vi "Filter Triggered.vi"(8 "error in (no error)":errorcluster, 10 "Assert Message":T1, 11 "Boolean Filter in":refnum<class "Boolean Filter.lvclass">) -> (0 "error out":errorcluster, 2 "Filtered":bool)   [LabVIEW 2018, in "Assert API Components.lvlib" / "Boolean Filter.lvclass"]
uses:
  Boolean Filter.lvclass
  Message Data.ctl
  Failure Actions.ctl
  Base Filter.lvclass
  Assert API Components.lvlib
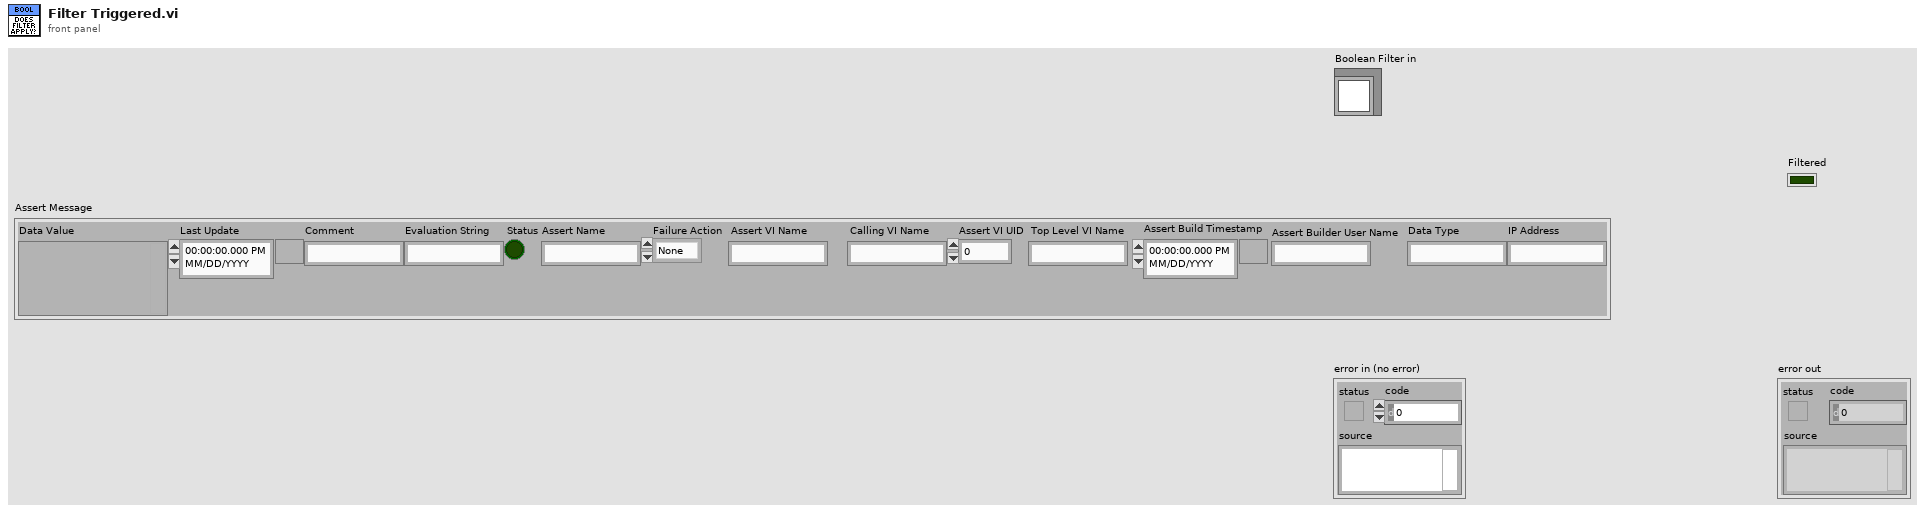
[diagram p1: front panel]
types:
  T1 = typedef "Assert API Components.lvlib/Message Data.ctl" = cluster{"Data Value":variant, "Last Update":timestamp, "Comment":string, "Evaluation String":string, "Status":bool, "Assert Name":string, "Failure Action":T2, "Assert VI Name":string, "Calling VI Name":string, "Assert VI UID":i32, "Top Level VI Name":string, "Assert Build Timestamp":timestamp, "Assert Builder User Name":string, "Data Type":string, "IP Address":string}
  T2 = typedef "Assert API Components.lvlib/Failure Actions.ctl" = enum16{"None", "Log To File", "Pause Execution", "Abort Execution"}
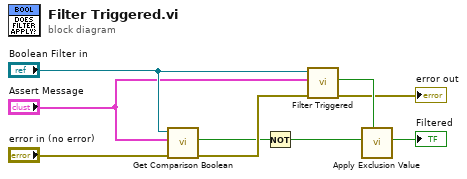
[diagram p0: block diagram]
diagram:
  n1 = call-dynamic "Get Comparison Boolean.vi"("error in (no error)"="error in (no error)", "Assert Message"="Assert Message", "Boolean Filter in"="Boolean Filter in") -> ("error out"=w9:errorcluster, "Comparison Value"=w8:bool)  [unwired: 7 in]
  n2 = Not(x=w8) -> (.not. x?=w7:bool)
  n3 = call-parent "Filter Triggered.vi"("error in (no error)"=w9, "Assert Message"="Assert Message", "Base Filter in"="Boolean Filter in") -> ("error out"=→"error out":errorcluster, "Filtered"=w6:bool)  [unwired: 7 in]
  n4 = call "Apply Exclusion Value.vi"("Excluded?"=w6, "Filtered value in"=w7) -> ("Final Filtered Value"=→"Filtered":bool)  [unwired: 9 in]
